vi "folder_creation.vi"(1 "Name":string) -> (0 "String":string)   [LabVIEW 2015]
doc: "This VI creates a folder of a following type: Prename_dd_mm_yyyy. Prename is configure on the Front Panel of the main VI. If the folder with the generated name already exists, the new folder is not created."
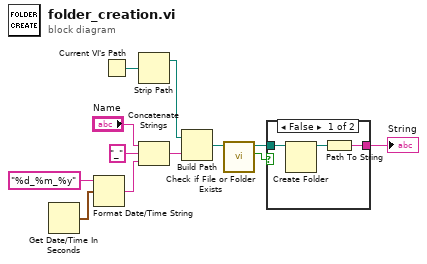
[diagram p0: block diagram]
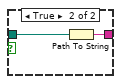
[diagram p2: hidden frame]
diagram:
  n1 = Get Date/Time In Seconds() -> (seconds since 1Jan1904=w11:timestamp)
  n2 = Format Date/Time String(time format string (%c)="%d_%m_%y", seconds (now)=w11) -> (date/time string=w3:string)  [unwired: 1 in]
  n3 = Current VI's Path() -> (path=w12:path)
  n4 = Strip Path(path=w12) -> (stripped path=w9:path)  [unwired: 1 out]
  n5 = Concatenate Strings("Name", "_" ("string"), w3) -> (w2:string)
  n6 = Build Path(base path=w9, name or relative path=w2) -> (appended path=w1:path)
  n7 = call <vilib>:"Check if File or Folder Exists.vi"("path"=w1) -> ("file or folder exists?"=w8:bool, "dup path"=w7:path)  [unwired: 8 in, 1 out]
  n8 = case shown="False" w8 {
    tunnel: w7 -> [w15 w17]
    tunnel: [w13 w16] -> w6
    frame False {
      n9 = Create Folder(path (use dialog)=w15) -> (created path=w14:path)  [unwired: 2 in, 2 out]
      n10 = Path To String(path=w14) -> (string=w13:string)
    }
    frame True {
      n11 = Path To String(path=w17) -> (string=w16:string)
    }
  }
  "String" <- w6
